vi "SaveVi.vi"(8 "error in":errorcluster, 11 "State":T1) -> (0 "error out":errorcluster, 3 "State out":T1)   [LabVIEW 2013, in "data interface script.lvlib"]
uses:
  data interface script.lvlib
  Controls/StateCluster.ctl
  Controls/initialized references.ctl
  Controls/interface VI type.ctl
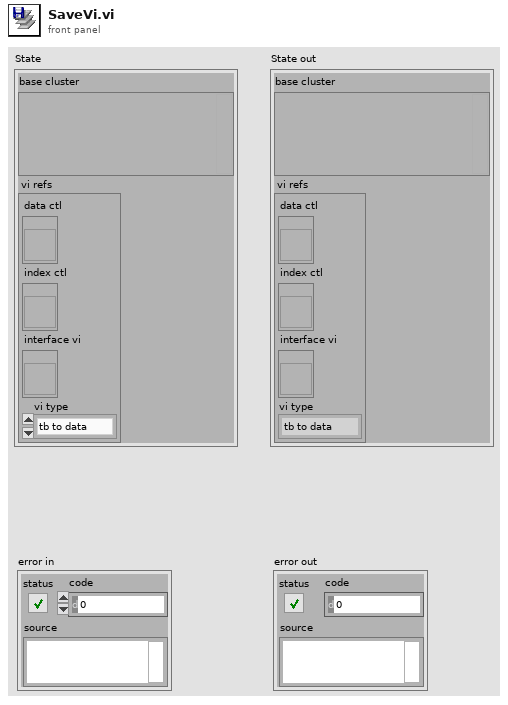
[diagram p1: front panel]
types:
  T1 = typedef "data interface script.lvlib/StateCluster.ctl" = cluster{"base cluster":variant, "vi refs":T2}
  T2 = typedef "data interface script.lvlib/initialized references.ctl" = cluster{"data ctl":refnum<vi>, "index ctl":refnum<vi>, "interface vi":refnum<vi>, "vi type":T3}
  T3 = typedef "data interface script.lvlib/interface VI type.ctl" = enum16{"tb to data", "data to tb"}
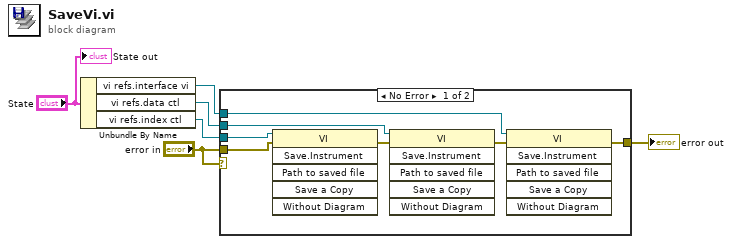
[diagram p0: block diagram]
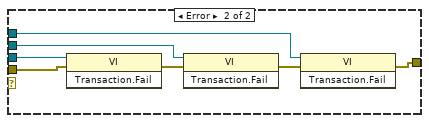
[diagram p2: hidden frame]
diagram:
  n1 = Unbundle By Name("State") -> ("vi refs.interface vi"=w6:refnum<vi>, "vi refs.data ctl"=w3:refnum<vi>, "vi refs.index ctl"=w2:refnum<vi>)
  n2 = case shown="No Error" "error in" {
    tunnel: w6 -> [w8 w16]
    tunnel: [w13 w17] -> w4
    tunnel: w3 -> [w9 w15]
    tunnel: w2 -> [w11 w14]
    tunnel: "error in" -> [w10 w20]
    frame No Error {
      n3 = invoke class="VI" method="Save.Instrument"(reference=w11, error in=w10) -> (error out=w7:errorcluster)  [unwired: 4 in, 5 out]
      n4 = invoke class="VI" method="Save.Instrument"(reference=w9, error in=w7) -> (error out=w12:errorcluster)  [unwired: 4 in, 5 out]
      n5 = invoke class="VI" method="Save.Instrument"(reference=w8, error in=w12) -> (error out=w13:errorcluster)  [unwired: 4 in, 5 out]
    }
    frame Error {
      n6 = invoke class="VI" method="Transaction.Fail"(reference=w14, error in=w20) -> (error out=w19:errorcluster)  [unwired: 1 in, 2 out]
      n7 = invoke class="VI" method="Transaction.Fail"(reference=w15, error in=w19) -> (error out=w18:errorcluster)  [unwired: 1 in, 2 out]
      n8 = invoke class="VI" method="Transaction.Fail"(reference=w16, error in=w18) -> (error out=w17:errorcluster)  [unwired: 1 in, 2 out]
    }
  }
  "error out" <- w4
  "State out" <- "State"
